vi "Project Robot Arm 2 (1).vi"() -> ()   [LabVIEW 2023]
uses:
  <vilib>/DAQmx/read.llb/DAQmx Read (Analog Wfm 1Chan NSamp).vi
  <vilib>/Analysis/baseanly.llb/Mean (DBL).vi
  <vilib>/DAQmx/create/channels.llb/DAQmx Create Channel (AI-Voltage-Basic).vi
  <vilib>/DAQmx/configure/timing.llb/DAQmx Timing (Sample Clock).vi
  <vilib>/DAQmx/miscellaneous.llb/DAQmx Fill In Error Info.vi
  <vilib>/measure/maspectr.llb/FFT Spectrum (Mag-Phase) for 1 Chan.vi
  <vilib>/measure/matone.llb/Extract Single Tone Information 1 Chan.vi
  <vilib>/measure/madcrms.llb/Basic Averaged DC-RMS for 1 Chan.vi
  <vilib>/Analysis/NI_AALBase.lvlib
  <vilib>/measure/NI_MAPro.lvlib
panel:
  out "Angle 1":dbl caption="Servo Angle 1"
  out "Position 1":i32 caption="Servo Position 1"
  out "RMS x Factor":dbl
  in  "Factor":dbl
  out "RMS value":dbl
  out "Best Frequency":dbl
  out "Waveform Graph 2":cluster{"f0":dbl, "df":dbl, "magnitude":dbl[]}(graph)
  in  "stop":bool
  in  "Sampling Frequency":dbl=1000.0
  in  "Samples per Channel":i32=100
  out "Waveform Graph":waveform(dbl)(graph)
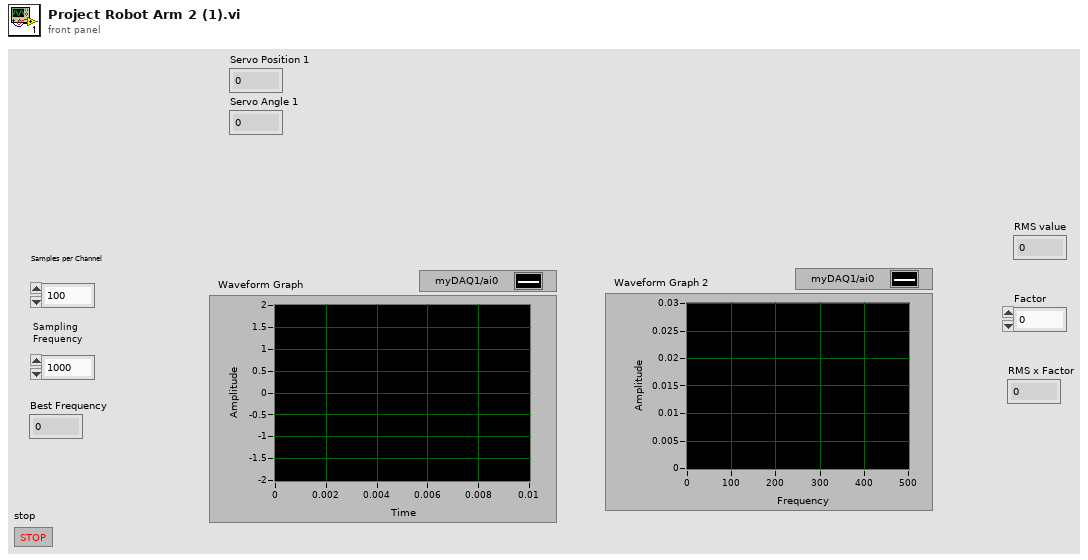
[diagram p1: front panel]
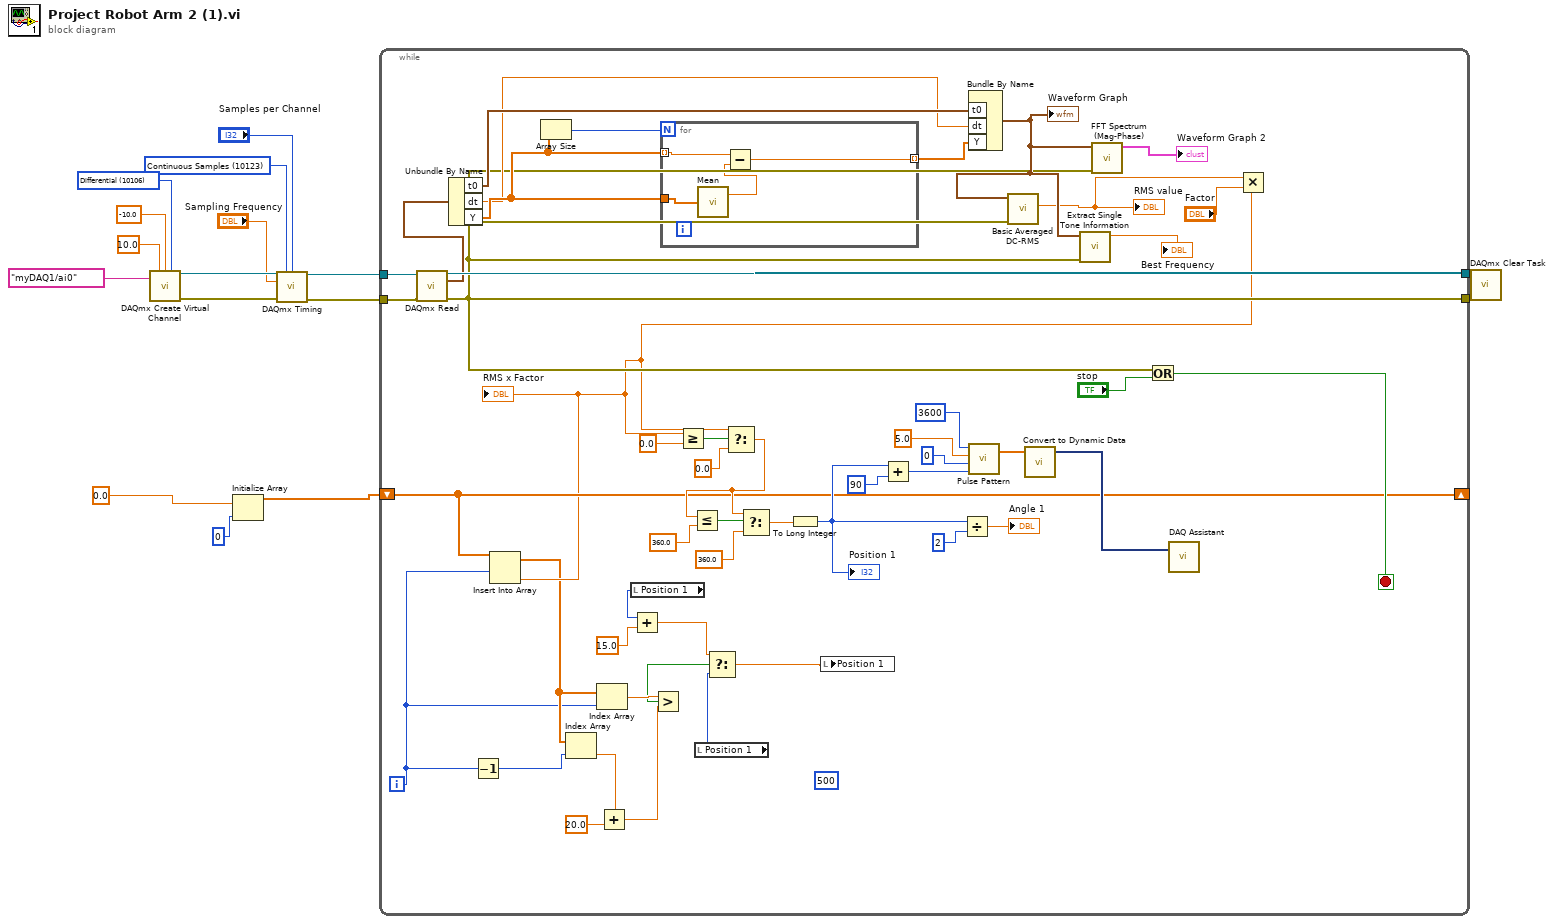
[diagram p0: block diagram]
diagram:
  w9 = 10123 items=["Finite Samples"=10178, "Continuous Samples"=10123, "Hardware Timed Single Point"=12522] ("sample mode")
  w13 = 10106 items=["Default"=-1, "RSE"=10083, "NRSE"=10078, "Differential"=10106, "Pseudodifferential"=12529] ("input terminal configuration")
  n1 = call-poly <vilib>:"DAQmx Create Virtual Channel.vi"("maximum value"=10.0, "minimum value"=-10.0, "input terminal configuration"=w13, "physical channels"=tag "myDAQ1/ai0") -> ("task out"=w12:refnum<k21>, "error out"=w11:errorcluster)  [unwired: 10 in]
  n2 = Initialize Array(0.0 ("element"), 0 ("dimension size")) -> (w1:dbl[])
  n3 = call-poly <vilib>:"DAQmx Timing.vi"("task/channels in"=w12, "sample mode"=w9, "samples per channel"="Samples per Channel", "rate"="Sampling Frequency", "error in"=w11) -> ("task out"=w7:refnum<k21>, "error out"=w6:errorcluster)  [unwired: 9 in]
  n4 = while {
    tunnel: w7 -> [w66]
    tunnel: w6 -> [w65]
    tunnel: [w64] -> w5
    tunnel: [w54] -> w4
    shift-right: [w31] -> _
    shift-left: w1 -> [w31]
    i -> [w27]
    stop <- w52 stop-if-true
    (unwired) u32 500 ("milliseconds to wait")
    n5 = call-poly <vilib>:"DAQmx Read.vi"("task/channels in"=w66, "error in"=w65) -> ("task out"=w64:refnum<k21>, "data"=w63:waveform(dbl), "error out"=w54:errorcluster)  [unwired: 11 in]
    n6 = Unbundle By Name(w63) -> ("t0"=w59:timestamp, "dt"=w58:dbl, "Y"=w61:dbl[])
    n7 = Decrement(x=w27) -> (x-1=w26:i32)
    n8 = Array Size(array=w61) -> (size(s)=w62:i32)
    n9 = local read "Position 1"() -> (w24:i32)
    n10 = Add(x=w24, y=15.0) -> (x+y=w22:dbl)
    n11 = for {
      N: w62 -> [_]
      tunnel: [w70] -> w57 mode=indexing
      tunnel: w61 -> [w69] mode=indexing
      tunnel: w61 -> [w68]
      n12 = call-poly <vilib>:"Mean.vi"("X"=w68) -> ("mean"=w67:dbl)  [unwired: 1 out]
      n13 = Subtract(x=w69, y=w67) -> (x-y=w70:dbl)
    }
    n14 = local read "Position 1"() -> (w21:i32)
    n15 = Bundle By Name("t0"=w59, "dt"=w58, "Y"=w57) -> (w56:waveform(dbl))  [unwired: 1 in]
    "Waveform Graph" <- w56
    n16 = call-poly <vilib>:"Basic Averaged DC-RMS.vi"("error in (no error)"=w54, "signal in"=w56) -> ("RMS value"=w51:dbl)  [unwired: 6 in, 3 out]
    "RMS value" <- w51
    n17 = call-poly <vilib>:"Extract Single Tone Information.vi"("error in (no error)"=w54, "time signal in"=w56) -> ("detected frequency"=→"Best Frequency":dbl)  [unwired: 4 in, 5 out]
    n18 = call-poly <vilib>:"FFT Spectrum (Mag-Phase).vi"("error in (no error)"=w54, "time signal"=w56) -> ("magnitude"=→"Waveform Graph 2":cluster{"f0":dbl, "df":dbl, "magnitude":dbl[]})  [unwired: 5 in, 4 out]
    n19 = Or(x=w54, y="stop") -> (x .or. y?=w52:bool)
    n20 = Multiply(x=w51, y="Factor") -> (x*y=w30:dbl)
    "RMS x Factor" <- w30
    n21 = Insert Into Array(array=w31, index=w27, new element=w30) -> (w28:dbl[])
    n22 = Index Array(array=w28, index=w26) -> (element=w18:dbl)
    n23 = Index Array(array=w28, index=w27) -> (element=w29:dbl)
    n24 = Add(x=w18, y=20.0) -> (x+y=w17:dbl)
    n25 = Greater?(x=w29, y=w17) -> (0:w25:bool)
    n26 = Greater Or Equal?(x=w30, y=0.0) -> (x >= y?=w38:bool)
    n27 = Select(t=w22, s=w25, f=w21) -> (s? t:f=w20:dbl)
    n28 = Select(t=w30, s=w38, f=0.0) -> (s? t:f=w35:dbl)
    n29 = Less Or Equal?(x=w35, y=360.0) -> (x <= y?=w42:bool)
    n30 = Select(t=w35, s=w42, f=360.0) -> (s? t:f=w39:dbl)
    n31 = To Long Integer(number=w39) -> (32bit integer=w34:i32)
    "Position 1" <- w34
    n32 = local write "Position 1"(w20) -> ()
    n33 = Add(x=w34, y=90) -> (x+y=w45:i32)
    n34 = Divide(x=w34, y=2) -> (x/y=→"Angle 1":dbl)
    n35 = call <vilib>:"Pulse Pattern.vi"("width"=w45, "delay"=0, "amplitude"=5.0, "samples"=3600) -> ("Pulse Pattern"=w49:dbl[])  [unwired: 1 out]
    n36 = call "Convert to Dynamic Data"("Array"=w49) -> ("Dynamic Data Type"=w32:dynamicdata)  [unwired: 3 in]
    n37 = call "DAQ Assistant"("data"=w32) -> ()  [unwired: 16 in, 3 out]
  }
  n38 = call <vilib>:"DAQmx Clear Task.vi"("task in"=w5, "error in"=w4) -> ()  [unwired: 13 in, 1 out]
